vi "Write SequenceIndexName.vi"(8 "error in (no error)":errorcluster, 10 "SequenceIndexName":string, 11 "SequenceIndex in":refnum<class "SequenceIndex.lvclass">) -> (0 "error out":errorcluster, 3 "SequenceIndex out":refnum<class "SequenceIndex.lvclass">)   [LabVIEW 2013, in "SequenceIndex.lvclass"]
uses:
  SequenceIndex.lvclass
  SequenceIndex.lvclass/SequenceIndex.ctl
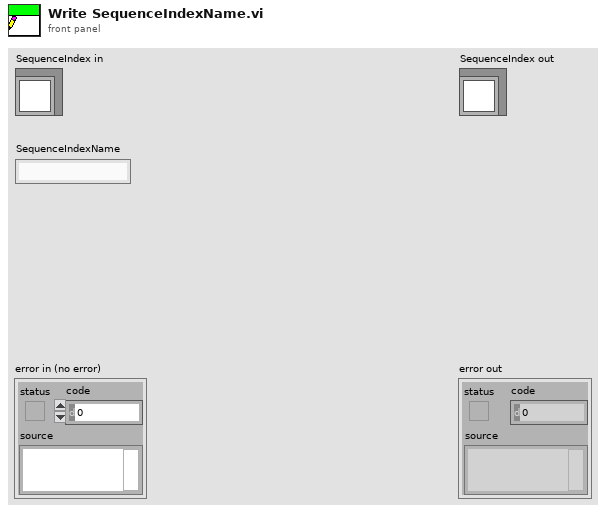
[diagram p1: front panel]
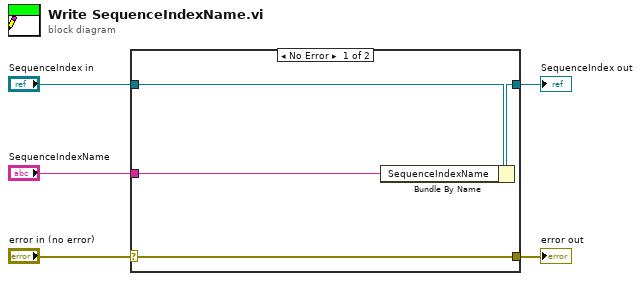
[diagram p0: block diagram]
diagram:
  n1 = case shown="No Error" "error in (no error)" {
    selector: "error in (no error)" -> [w9 w10]
    tunnel: [w9 w10] -> w4
    tunnel: [w7 w11] -> w2
    tunnel: "SequenceIndex in" -> [w8 w11]
    tunnel: "SequenceIndexName" -> [w6 _]
    frame No Error {
      n2 = Bundle By Name(cluster=w8, "SequenceIndexName"=w6) -> (w7:refnum<class "SequenceIndex.lvclass">)
    }
    frame Error {
    }
  }
  "error out" <- w4
  "SequenceIndex out" <- w2
